vi "timetest6.vi"() -> ()   [LabVIEW 2015]
uses:
  BERTTA.dll
panel:
  in  "Tcurrent":dbl
  in  "Tset":dbl=100.0
  out "double precision float":dbl
  out "element 7":i32
  out "return type":dbl
  in  "direction":i32
  out "element 6":i32
  in  "rt":i32=60
  out "element 5":i32
  out "element 3":i32
  out "element 2":i32
  out "element":i32
  in  "pause":i32
  in  "start":i32
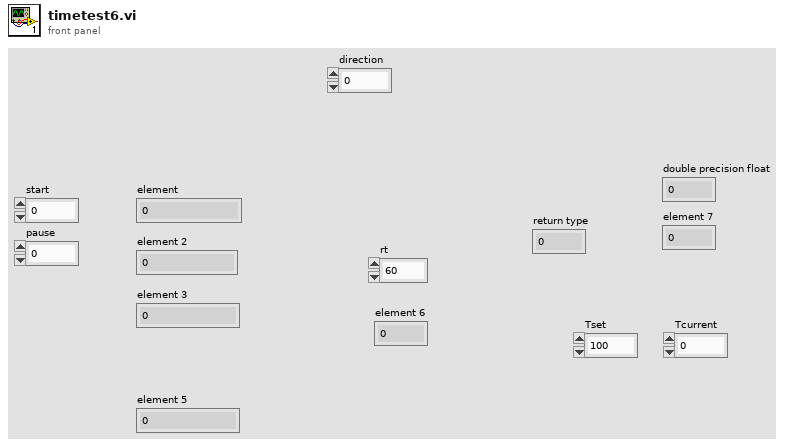
[diagram p1: front panel]
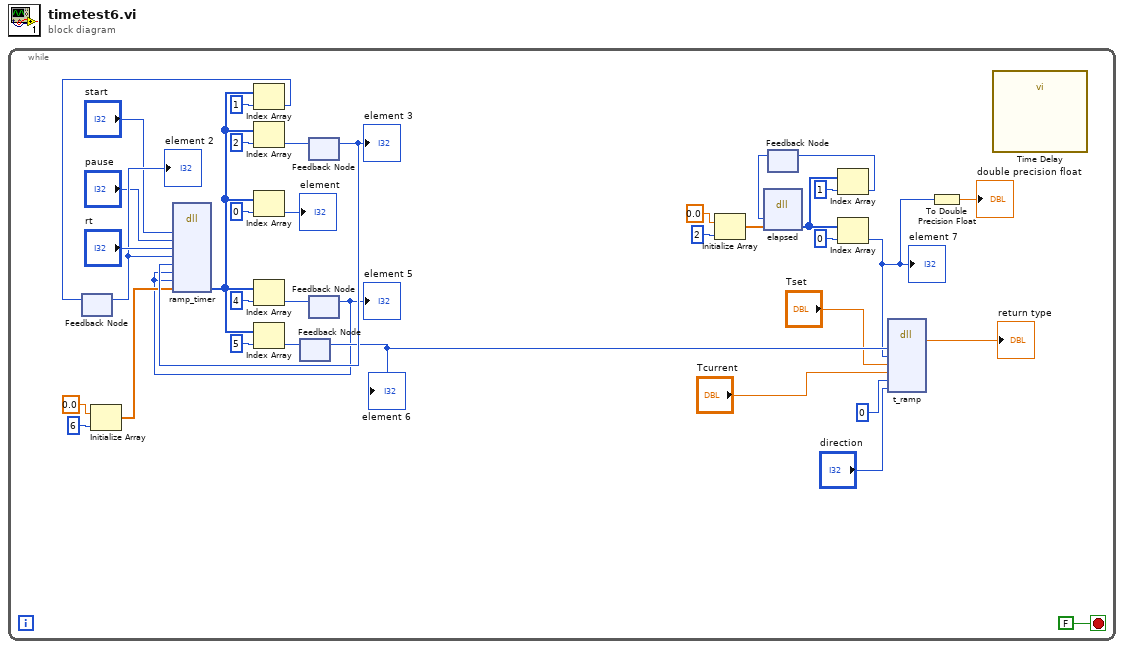
[diagram p0: block diagram]
diagram:
  n1 = while {
    stop <- FALSE stop-if-true
    n2 = feedback #1() -> (w29:i32)  [unwired: 1 in]
    "element 2" <- w29
    n3 = Initialize Array(0.0 ("element"), 6 ("dimension size")) -> (w21:dbl[])
    n4 = feedback #2() -> ()  [unwired: 2 in]
    n5 = feedback #3() -> (w31:i32)  [unwired: 1 in]
    "element 3" <- w31
    n6 = feedback #4() -> (w1:i32)  [unwired: 1 in]
    "element 5" <- w1
    n7 = dll-call lib="C:/Users/xlaraser/Documents/Visual Studio 2017/Projects/Bertta/BERTTA/Debug/BERTTA.dll" fn="ramp_timer"("enable"="start", "pause"="pause", "rt"="rt", "start_time"=w29, "pause_time"=w31, "paused"=w1, "paused_old"=w1, "params"=w21) -> ("params"=w36:i32[])  [unwired: 11 in, 2 out]
    n8 = Index Array(array=w36, index=1) -> (element=w28:i32)
    n9 = feedback-in #1(w28) -> ()
    n10 = Index Array(array=w36, index=2) -> (element=w30:i32)
    n11 = Index Array(array=w36, index=0) -> (element=→"element":i32)
    n12 = Index Array(array=w36, index=4) -> (element=w33:i32)
    n13 = Index Array(array=w36, index=5) -> (element=w8:i32)
    "element 6" <- w8
    n14 = feedback-in #2(w8) -> ()
    n15 = feedback-in #3(w30) -> ()
    n16 = feedback-in #4(w33) -> ()
    n17 = Initialize Array(0.0 ("element"), 2 ("dimension size")) -> (w16:dbl[])
    n18 = feedback #5() -> (w9:i32)  [unwired: 1 in]
    n19 = dll-call lib="C:/Users/xlaraser/Documents/Visual Studio 2017/Projects/Bertta/BERTTA/Debug/BERTTA.dll" fn="elapsed"("last_time"=w9, "params"=w16) -> ("params"=w12:i32[])  [unwired: 5 in, 2 out]
    n20 = Index Array(array=w12, index=1) -> (element=w10:i32)
    n21 = feedback-in #5(w10) -> ()
    n22 = Index Array(array=w12, index=0) -> (element=w6:i32)
    "element 7" <- w6
    n23 = dll-call lib="C:/Users/xlaraser/Documents/Visual Studio 2017/Projects/Bertta/BERTTA/Debug/BERTTA.dll" fn="t_ramp"("ramp_time"=w8, "elapsed"=w6, "Tset"="Tset", "Tcurrent"="Tcurrent", "rt"=0, "direction"="direction") -> ("return type"=→"return type":dbl)  [unwired: 9 in, 2 out]
    n24 = To Double Precision Float(number=w6) -> (double precision float=→"double precision float":dbl)
    n25 = call "Time Delay"() -> ()  [unwired: 11 in, 1 out]
  }
